vi "FRCts20_Backend_INI_Read_Competition.vi"(8 "error in (no error)":errorcluster, 11 "INI Controller in":refnum<class "FRCts20_Backend_INI Controller.lvclass">) -> (0 "error out":errorcluster, 2 "Competition Name":string, 3 "INI Controller out":refnum<class "FRCts20_Backend_INI Controller.lvclass">)   [LabVIEW 2013, in "FRCts20_Backend_Engine.lvlib" / "FRCts20_Backend_INI Controller.lvclass"]
uses:
  FRCts20_Backend_INI Controller.lvclass
  FRCts20_Backend_INI Controller.lvclass/FRCts20_Backend_INI Controller.ctl
  <vilib>/Utility/config.llb/Read Key (String).vi
  <vilib>/Utility/config.llb/NI_LVConfig.lvlib
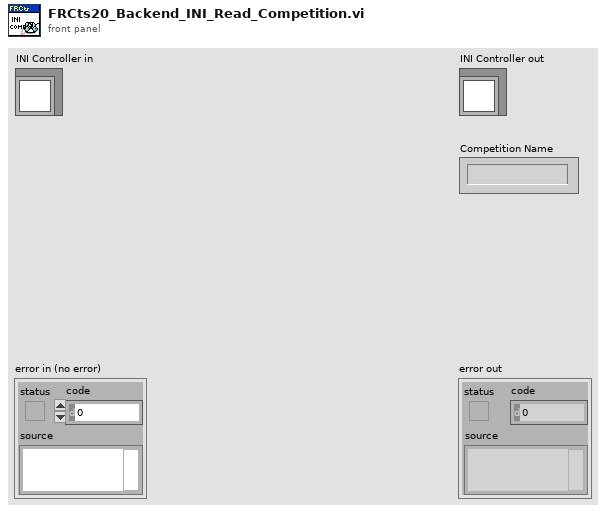
[diagram p1: front panel]
types:
  T1 = typedef "NI_LVConfig.lvlib/Config Data RefNum.ctl" = refnum<k1>
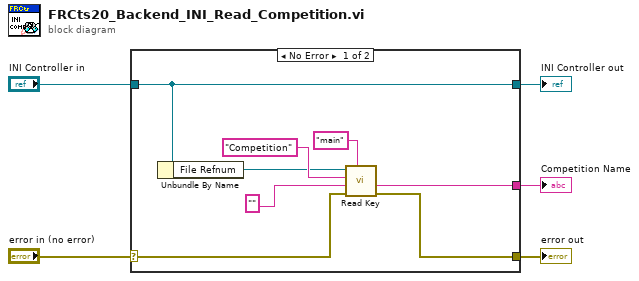
[diagram p0: block diagram]
diagram:
  n1 = case shown="No Error" "error in (no error)" {
    selector: "error in (no error)" -> [w7 w14]
    tunnel: [w8 w14] -> w4
    tunnel: [w13 w15] -> w2
    tunnel: "INI Controller in" -> [w13 w15]
    tunnel: [w9 _] -> w1
    frame No Error {
      n2 = Unbundle By Name(w13) -> ("File Refnum"=w11:T1)
      n3 = call-poly <vilib>:"Read Key.vi"("section"="main", "error in (no error)"=w7, "default value"="", "key"="Competition", "refnum"=w11) -> ("error out"=w8:errorcluster, "value"=w9:string)  [unwired: 3 in, 2 out]
    }
    frame Error {
    }
  }
  "error out" <- w4
  "INI Controller out" <- w2
  "Competition Name" <- w1
